vi "Vision Main.vi"(11 "Camera Image":T2(plugin-control)) -> ()   [LabVIEW 2012]
panel:
  out "Particle Reports (Pixels)":T1(array[cluster]) {"Orientation" format="%.2f"; "Dimensions"."Height" format="%.2f"; "Dimensions"."Width" format="%.2f"; "Center of Mass"."Y" format="%.2f"; "Center of Mass"."X" format="%.2f"; "Bounding Rect"."Bottom" format="%.2f"; "Bounding Rect"."Right" format="%.2f"; "Bounding Rect"."Top" format="%.2f"; "Bounding Rect"."Left" format="%.2f"; "Number of Holes" format="%.2f"; "Area" format="%.2f"}
  out "Number of Particles":i32
  out "Processed Image":T2(plugin-control)
  out "Cropped Image":T2(plugin-control)
  # "Camera Image"
  # "diffrence from center, rectangle mojo"
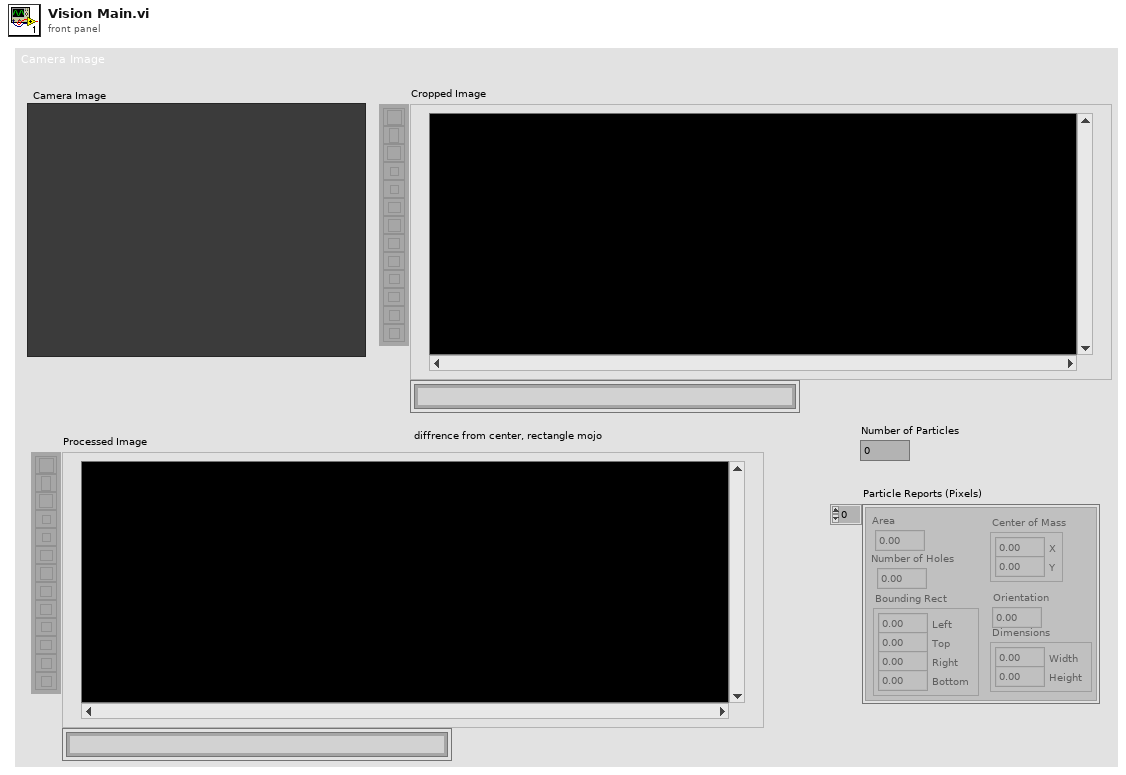
[diagram p1: front panel]
types:
  T1 = cluster{"Area":dbl, "Number of Holes":dbl, "Bounding Rect":cluster{"Left":dbl, "Top":dbl, "Right":dbl, "Bottom":dbl}, "Center of Mass":cluster{"X":dbl, "Y":dbl}, "Orientation":dbl, "Dimensions":cluster{"Width":dbl, "Height":dbl}}[]
  T2 = typedef "IMAQ Image.ctl" = refnum<image>
  T3 = typedef "Image Type" = u32
  T4 = cluster{"Area":dbl, "Number of Holes":dbl, "Bounding Rect":cluster{"Left":dbl, "Top":dbl, "Right":dbl, "Bottom":dbl}, "Center of Mass":cluster{"X":dbl, "Y":dbl}, "Orientation":dbl, "Dimensions":cluster{"Width":dbl, "Height":dbl}, "Rectangle Mojo":dbl, "Distance":dbl, "Location X":dbl, "Angle":dbl}[]
  T5 = cluster{"Area":dbl, "Number of Holes":dbl, "Bounding Rect":cluster{"Left":dbl, "Top":dbl, "Right":dbl, "Bottom":dbl}, "Center of Mass":cluster{"X":dbl, "Y":dbl}, "Orientation":dbl, "Dimensions":cluster{"Width":dbl, "Height":dbl}, "Rectangle Mojo":dbl, "Distance":dbl, "Location X":dbl, "Angle":dbl}
  T6 = cluster{"Left":i32, "Top":i32, "Right":i32, "Bottom":i32}
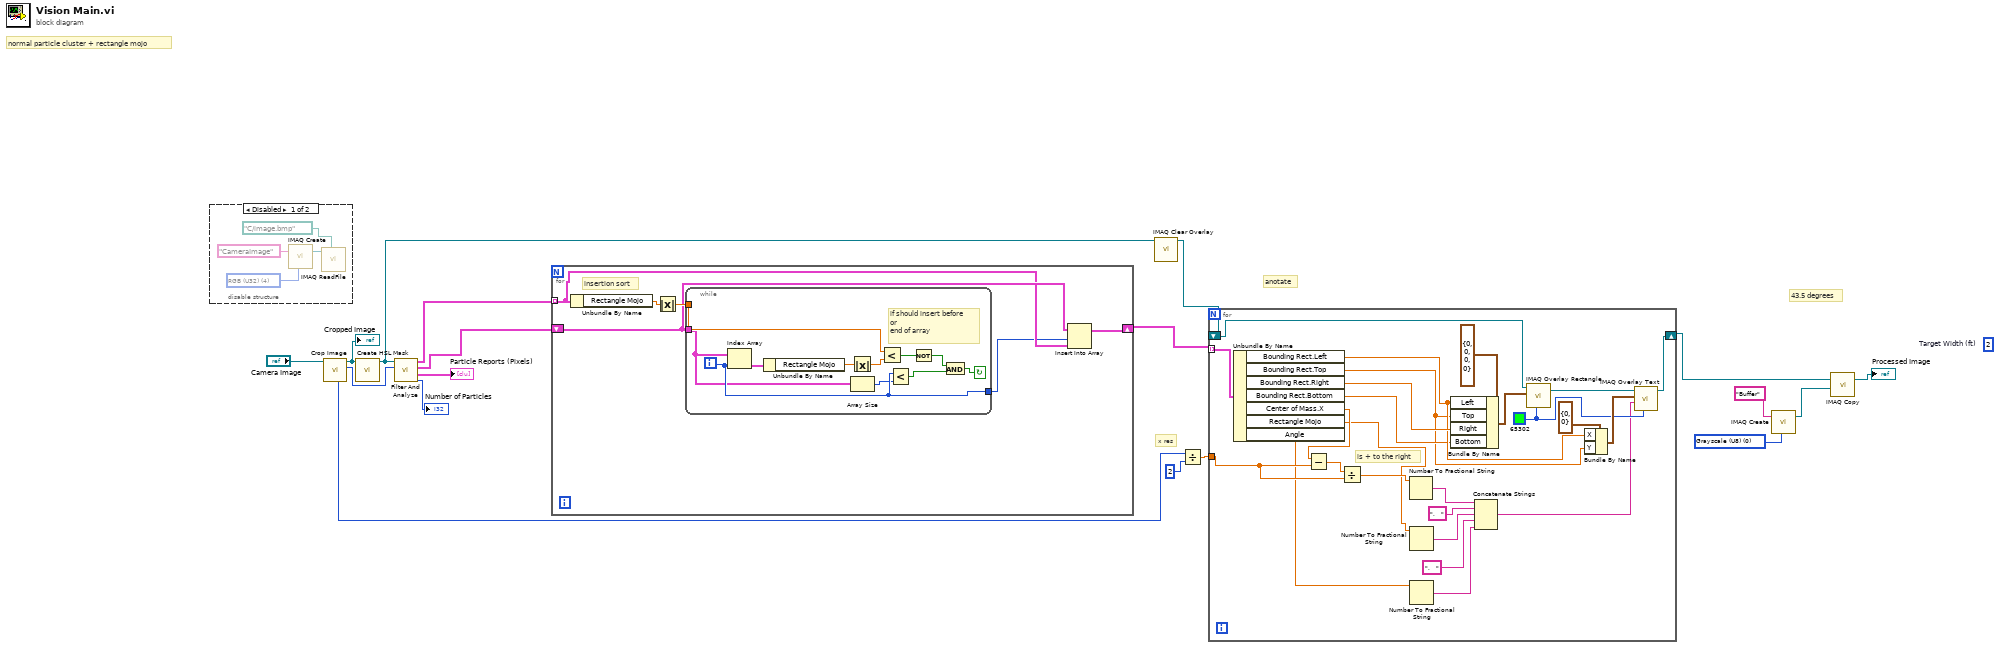
[diagram p0: block diagram]
diagram:
  (unwired) 2  # Target Width (ft)
  w13 = T3 0 items=["Grayscale (U8)", "Grayscale (I16)", "Grayscale (SGL)", "Complex (CSG)", "RGB (U32)", "HSL (U32)", "RGB (U64)", "Grayscale (U16)"] ("Image Type")
  # "43.5 degrees"
  # "x res"
  # "normal particle cluster + rectangle mojo"
  # "anotate"
  n1 = disable-structure shown="Disabled" {
    frame Disabled {
      w20 = T3 4 items=["Grayscale (U8)", "Grayscale (I16)", "Grayscale (SGL)", "Complex (CSG)", "RGB (U32)", "HSL (U32)", "RGB (U64)", "Grayscale (U16)"] ("Image Type")
      n2 = call "IMAQ Create"("Image Name"="CameraImage", "Image Type"=w20) -> ("New Image"=w23:T2)  [unwired: 3 in, 1 out]
      n3 = call "IMAQ ReadFile"("File Path"=path "C:/image.bmp", "Image"=w23) -> ("Image Out"=w19:T2)  [unwired: 5 in, 4 out]
    }
    frame Enabled {
    }
  }
  n4 = call "Crop Image.vi"("Camera Image"="Camera Image") -> ("Y Resolution"=w6:i32, "Cropped Image"=w17:T2, "X Resolution"=w1:i32)  [unwired: 8 in]
  "Cropped Image" <- w17
  n5 = call "Create HSL Mask.vi"("Cropped Image"=w17) -> ("Image Mask"=w10:T2)  [unwired: 10 in]
  n6 = call "Filter And Analyze.vi"("Y Resolution"=w6, "Refnum in"=w10) -> ("Number of Particles"=→"Number of Particles":i32, "Particle Reports (Pixels)"=→"Particle Reports (Pixels)":T1, "Empty Array"=w4:T4, "Filtered Array"=w5:T4)  [unwired: 6 in]
  n7 = for {
    tunnel: w5 -> [w26] mode=indexing
    shift-right: [w25] -> w7
    shift-left: w4 -> [w27]
    # "insertion sort"
    n8 = Unbundle By Name(w26) -> ("Rectangle Mojo"=w29:dbl)
    n9 = Absolute Value(x=w29) -> (abs(x)=w28:dbl)
    n10 = while {
      tunnel: w27 -> [w35]
      tunnel: w28 -> [w38]
      tunnel: [w36] -> w24
      i -> [w36]
      stop <- w33 continue-if-true
      # "if should insert before\nor\nend of array"
      n11 = Index Array(array=w35, index=w36) -> (element=w40:T5)
      n12 = Unbundle By Name(w40) -> ("Rectangle Mojo"=w39:dbl)
      n13 = Absolute Value(x=w39) -> (abs(x)=w37:dbl)
      n14 = Array Size(array=w35) -> (size(s)=w34:i32)
      n15 = Less?(x=w38, y=w37) -> (x < y?=w31:bool)
      n16 = Less?(x=w36, y=w34) -> (x < y?=w32:bool)
      n17 = Not(x=w31) -> (.not. x?=w30:bool)
      n18 = And(x=w30, y=w32) -> (x .and. y?=w33:bool)
    }
    n19 = Insert Into Array(array=w27, index=w24, new element=w26) -> (w25:T4)
  }
  n20 = call "IMAQ Clear Overlay"("Image"=w10) -> ("Image Out"=w9:T2)  [unwired: 9 in, 1 out]
  n21 = Divide(x=w1, y=2) -> (x/y=w15:dbl)
  n22 = for {
    tunnel: w15 -> [w53]
    tunnel: w7 -> [w51] mode=indexing
    shift-right: [w45] -> w11
    shift-left: w9 -> [w44]
    w56 = u32 65302 ("Color")
    # "is + to the right"
    n23 = Unbundle By Name(w51) -> ("Bounding Rect.Left"=w59:dbl, "Bounding Rect.Top"=w57:dbl, "Bounding Rect.Right"=w63:dbl, "Bounding Rect.Bottom"=w58:dbl, "Center of Mass.X"=w55:dbl, "Rectangle Mojo"=w50:dbl, "Angle"=w41:dbl)
    n24 = Subtract(x=w55, y=w53) -> (x-y=w54:dbl)
    n25 = Divide(x=w54, y=w53) -> (x/y=w52:dbl)
    n26 = Number To Fractional String(number=w52) -> (F-format string=w49:string)  [unwired: 3 in]
    n27 = Number To Fractional String(number=w50) -> (F-format string=w47:string)  [unwired: 3 in]
    n28 = Number To Fractional String(number=w41) -> (F-format string=w42:string)  [unwired: 3 in]
    n29 = Bundle By Name(cluster=T6 {"Left"=0, "Top"=0, "Right"=0, "Bottom"=0} ("Rectangle"), "Left"=w59, "Top"=w57, "Right"=w63, "Bottom"=w58) -> (w64:T6)
    n30 = Concatenate Strings(w49, ",   ", w47, ",   ", w42) -> (w46:string)
    n31 = call "IMAQ Overlay Rectangle"("Color"=w56, "Rectangle"=w64, "Image"=w44) -> ("Image Out"=w62:T2)  [unwired: 3 in, 5 out]
    n32 = Bundle By Name(cluster=cluster{"X":i32, "Y":i32} {"X"=0, "Y"=0} ("Origin"), "X"=w59, "Y"=w57) -> (w60:cluster{"X":i32, "Y":i32})
    n33 = call "IMAQ Overlay Text"("Text Color (black)"=w56, "String"=w46, "Origin"=w60, "Image"=w62) -> ("Image Out"=w45:T2)  [unwired: 6 in, 1 out]
  }
  n34 = call "IMAQ Create"("Image Name"="Buffer", "Image Type"=w13) -> ("New Image"=w14:T2)  [unwired: 3 in, 1 out]
  n35 = call "IMAQ Copy"("Image Dst"=w14, "Image Src"=w11) -> ("Image Dst Out"=→"Processed Image":T2)  [unwired: 4 in, 1 out]
